vi "RT Main.vi"() -> ()   [LabVIEW 2011]
uses:
  RT/TypeDefs/Recipe Engine Commands.ctl
  RT/TypeDefs/Recipe Engine States.ctl
  <vilib>/Platform/TimedLoop/XDataNode/timing_clust.ctl
  <vilib>/Platform/TimedLoop/XDataNode/nitl_modes.ctl
  <vilib>/Platform/TimedLoop/XDataNode/wakeup.ctl
  RT/TypeDefs/Recipe Phase.ctl
  <vilib>/FPGAPlugInAG/cRIO-9074/niLvFpga_Open_cRIO-9074.vi
  <vilib>/rvi/interface/common/dynamic/niFpgaDynamicAddResources.vi
  <vilib>/FPGAPlugInAG/Dynamic/niLvFpga_Close_Dynamic.vi
  <vilib>/Platform/TimedLoop/XDataNode/loadnilvce.vi
  <vilib>/addons/control/pid/pid.llb/PID (DBL).vi
  <vilib>/Platform/TimedLoop/XDataNode/XDataNode.xnode
  <vilib>/rvi/interface/nirviOpenFPGA/nirviOpenFPGA.xnode
  FPGA Bitfiles/Bioreactor_FPGATarget_FPGAMain_8731874D.lvbitx
  FPGA Main.vi
  <vilib>/rvi/interface/nirviCloseFPGA/nirviCloseFPGA.xnode
  <vilib>/addons/control/pid/NI_PID_pid.lvlib
  <vilib>/Platform/TimedLoop/XDataNode/XDNodeRunTimeDep.lvlib
panel:
  out "FPGA State":enum16{"Normal Operation", "Safe State"}(ring)
  out "error out":errorcluster
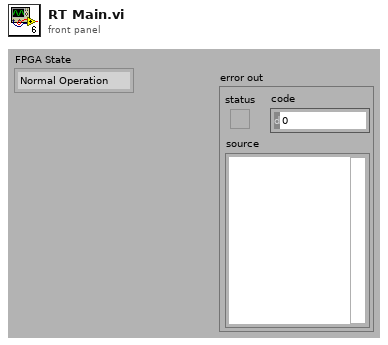
[diagram p1: front panel]
types:
  T1 = typedef "Recipe Engine Commands.ctl" = enum16{"Run Recipe", "Abort Recipe", "Exit"}
  T2 = typedef "Recipe Engine States.ctl" = enum16{"Initialize", "Wait for Cmd", "Load Phase", "Run Phase", "Exit"}
  T3 = typedef "XDNodeRunTimeDep.lvlib/timing_clust.ctl" = cluster{"Expected End [f-1]":u64, "Actual End [f-1]":u64, "Finished Late? [f-1]":bool, "Expected End [i-1]":u64, "Actual End [i-1]":u64, "Finished Late? [i-1]":bool, "Expected Start [i]":u64, "Actual Start [i]":u64, "Expected Start [f]":u64, "Actual Start [f]":u64, "Source Name":string, "Structure Name":string, "Period":i64, "Deadline":i64, "Offset":i64, "Start":i64, "Priority":i32, "Timeout":i32, "Mode":T4, "Wakeup Reason":T5, "Error":errorcluster, "Source Type":string, "Secondary Source Type":string, "Global End Time":u64, "Global Start Time":u64, "Frame Duration":u64, "Iteration Duration":u64, "Assigned CPU":i32, "I/O Scan Engine Mode":u32}
  T4 = typedef "XDNodeRunTimeDep.lvlib/nitl_modes.ctl" = enum32{"No Change", "Process missed periods, maintain original phase", "Discard missed periods, maintain original phase", "Process missed periods, ignore original phase", "Discard missed periods, ignore original phase"}
  T5 = typedef "XDNodeRunTimeDep.lvlib/wakeup.ctl" = enum32{"Normal", "Aborted", "Asynchronous wakeup", "Timing source error", "Timed loop error", "Timeout"}
  T6 = typedef "Recipe Phase.ctl" = cluster{"Temp Setpoint":dbl, "pH Setpoint":dbl, "Agitation ON":bool, "Intake ON":bool, "Waste ON":bool, "Time (s)":i32}
  T7 = cluster{"proportional gain (Kc)":dbl, "integral time (Ti, min)":dbl, "derivative time (Td, min)":dbl}
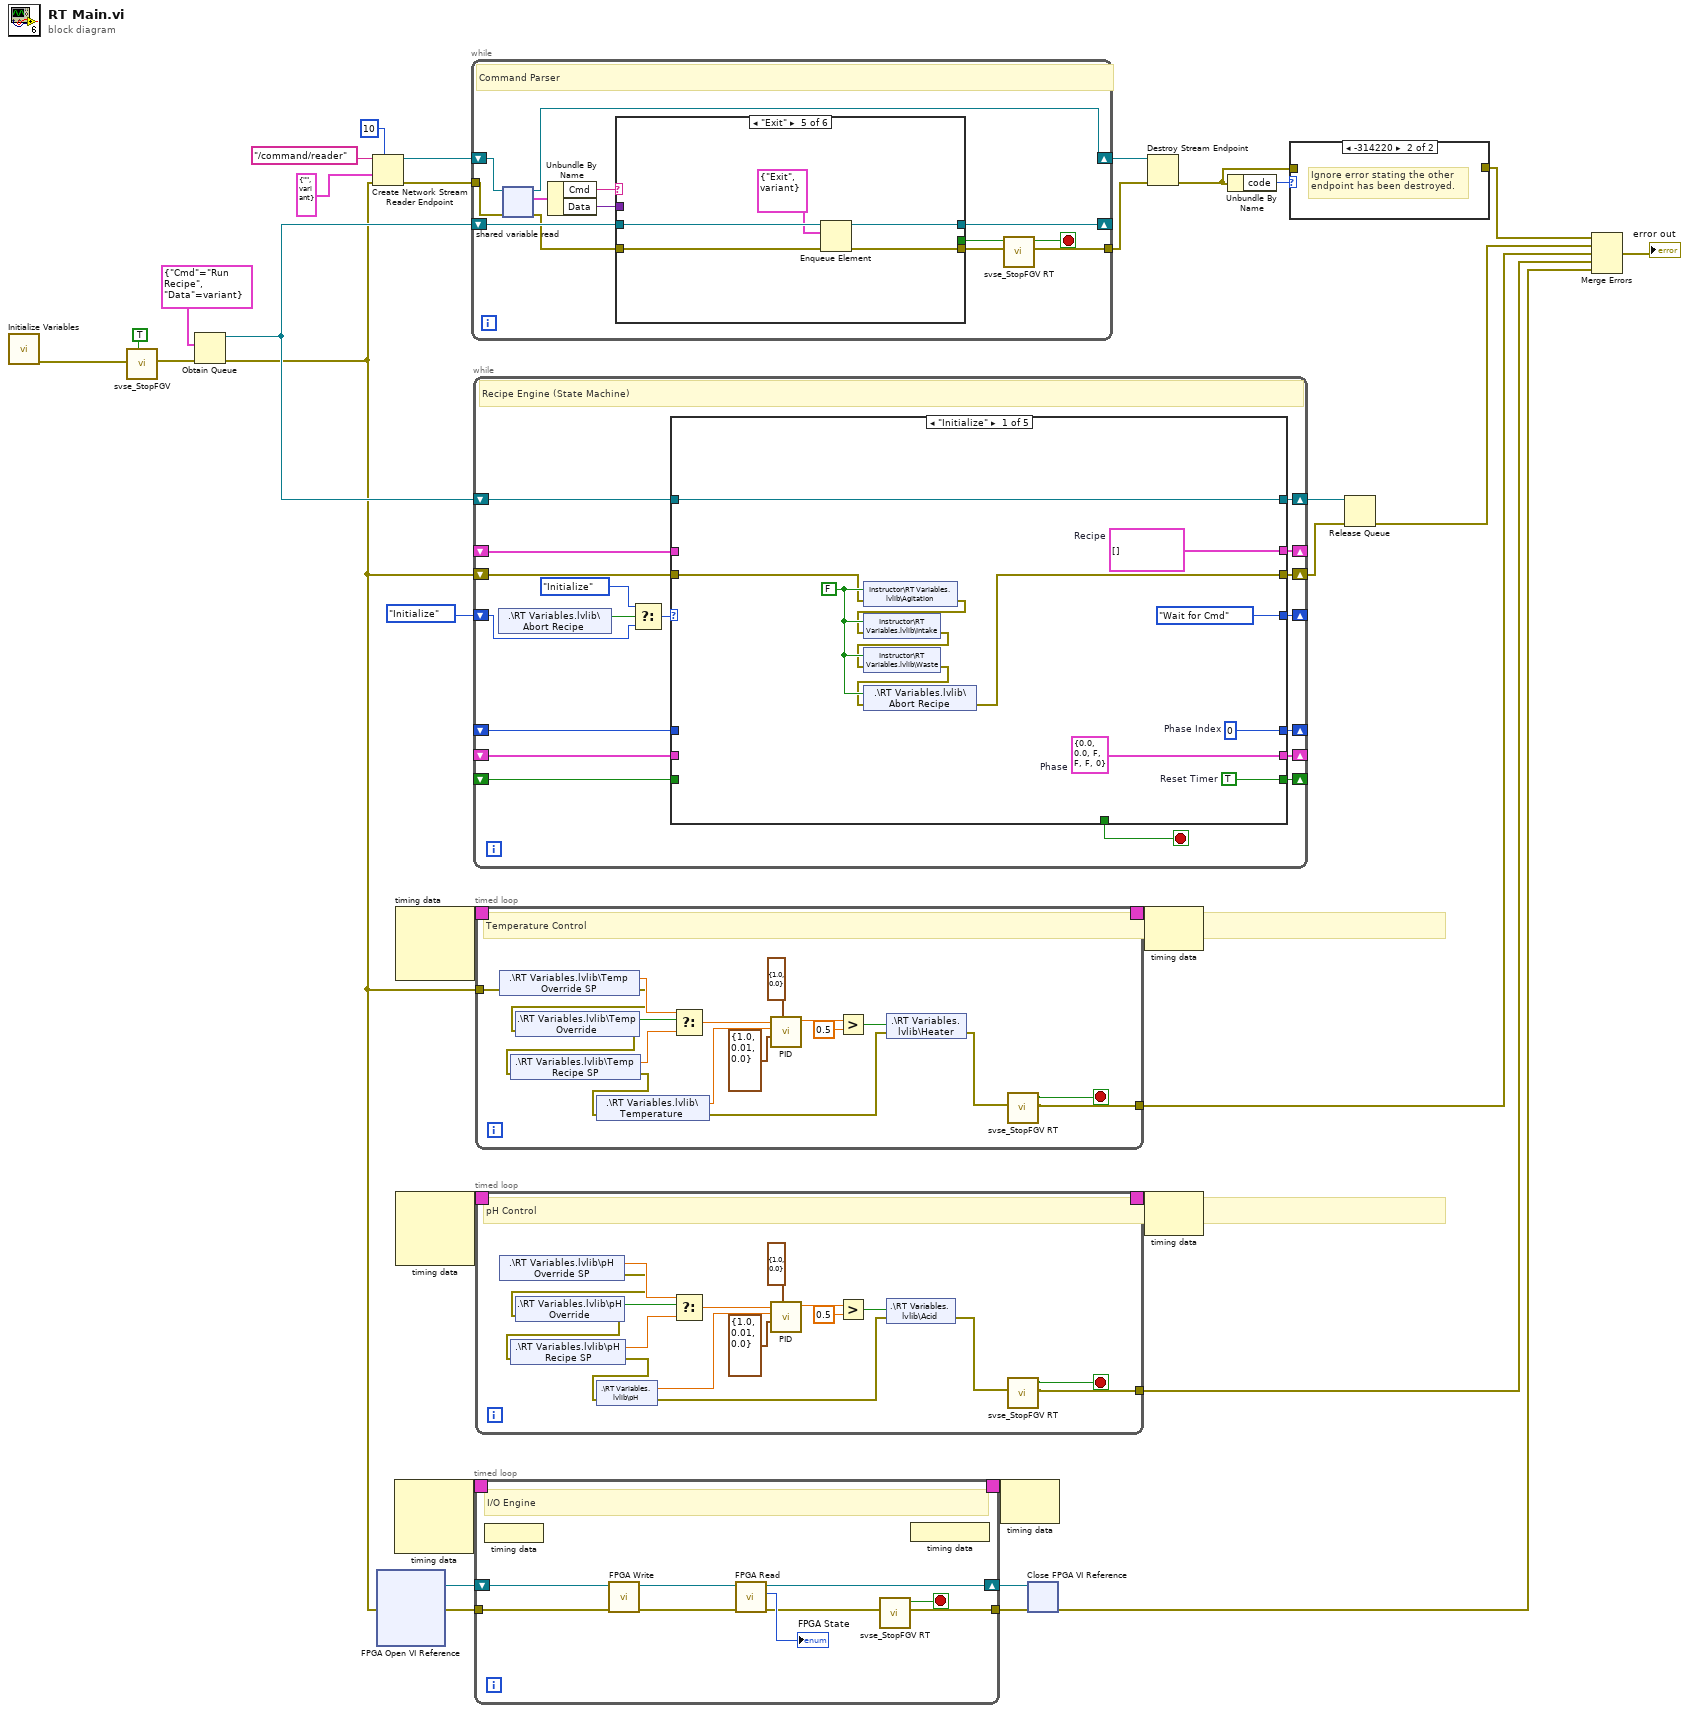
[diagram p0: block diagram]
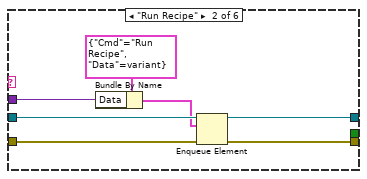
[diagram p4: hidden frame]
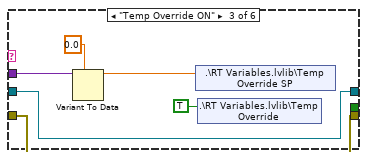
[diagram p5: hidden frame]
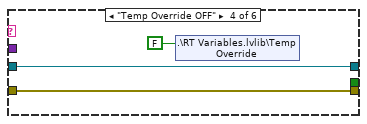
[diagram p6: hidden frame]
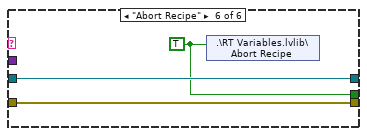
[diagram p7: hidden frame]
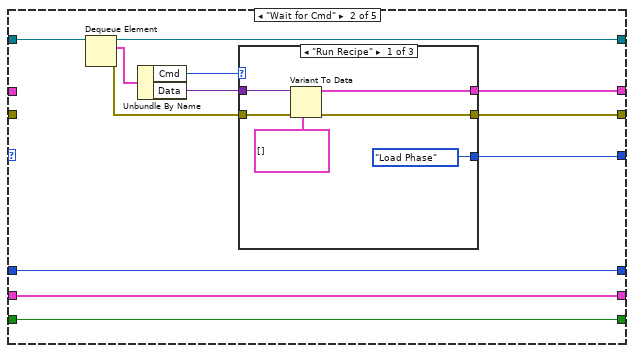
[diagram p8: hidden frame]
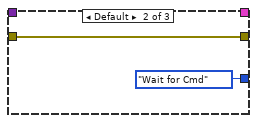
[diagram p9: hidden frame]
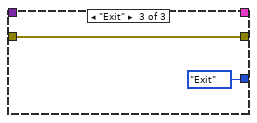
[diagram p10: hidden frame]
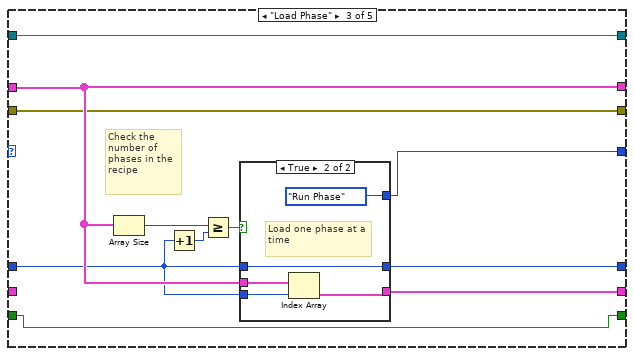
[diagram p11: hidden frame]
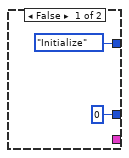
[diagram p12: hidden frame]
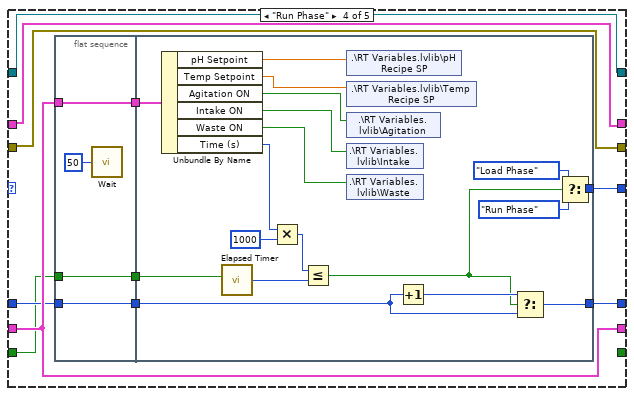
[diagram p13: hidden frame]
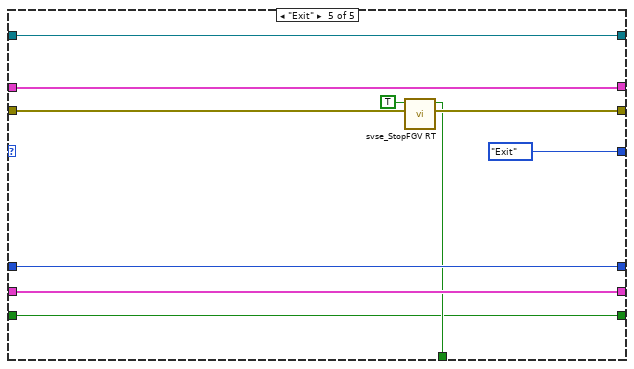
[diagram p14: hidden frame]
diagram:
  n1 = call "Initialize Variables.vi"() -> ("error out"=w9:errorcluster)  [unwired: 11 in]
  n2 = call "svse_StopFGV.vi"("Reset (F)"=TRUE, "error in"=w9) -> ("error out"=w8:errorcluster)  [unwired: 8 in, 1 out]
  n3 = Obtain Queue(element data type=cluster{"Cmd":T1, "Data":variant} {"Cmd"=enum."Run Recipe", "Data"=variant}, error in (no error)=w8) -> (queue out=w27:refnum<queue>, error out=w20:errorcluster)  [unwired: 3 in, 1 out]
  n4 = Create Network Stream Reader Endpoint(7:10 ("reader buffer size"), 8:w20, 9:cluster{"Cmd":string, "Data":variant} {"Cmd"="", "Data"=variant}, 11:"/command/reader" ("reader url")) -> (0:w28:errorcluster, 3:w30:refnum<k21>)  [unwired: 2 in]
  n5 = xnode "FPGA Open VI Reference"("error in"=w20) -> ("FPGA VI Reference Out"=w17:refnum<k20>, "error out"=w16:errorcluster)  [unwired: 1 in]
  n6 = node-c288() -> (w22:T3)  [unwired: 3 in]
  n7 = node-c288() -> (w26:T3)  [unwired: 3 in]
  n8 = node-c288() -> (w14:T3)  [unwired: 3 in]
  n9 = while {
    shift-right: [w35] -> w15
    shift-left: w30 -> [w43]
    shift-right: [w42] -> _
    shift-left: w27 -> [w44]
    tunnel: w28 -> [w41]
    tunnel: [w36] -> w4
    stop <- w38 stop-if-true
    # "Command Parser"
    n10 = shared-variable-read(w43, w41) -> (w35:refnum<k21>, w40:errorcluster, w47:cluster{"Cmd":string, "Data":variant})  [unwired: 1 in, 1 out]
    n11 = Unbundle By Name(w47) -> ("Cmd"=w46:string, "Data"=w45:variant)
    n12 = case shown="\"Exit\"" w46 {
      tunnel: w45 -> [_ w54 w62 _ _ _]
      tunnel: w44 -> [w49 w56 w60 w65 w70 w73]
      tunnel: [w49 w52 w60 w65 w68 w73] -> w42
      tunnel: w40 -> [w48 w51 w57 w63 w69 w72]
      tunnel: [w48 w50 w57 w63 w66 w72] -> w39
      tunnel: [_ _ _ _ _ w71] -> w37
      frame Default {
      }
      frame "Run Recipe" {
        n13 = Bundle By Name(cluster=cluster{"Cmd":T1, "Data":variant} {"Cmd"=enum."Run Recipe", "Data"=variant}, "Data"=w54) -> (w53:cluster{"Cmd":T1, "Data":variant})
        n14 = Enqueue Element(queue=w56, element=w53, error in (no error)=w51) -> (queue out=w52:refnum<queue>, error out=w50:errorcluster)  [unwired: 1 in, 1 out]
      }
      frame "Temp Override ON" {
        n15 = Variant To Data(type=0.0, Variant=w62) -> (data=w59:dbl)  [unwired: 1 in, 1 out]
        n16 = shared-variable ".\\RT Variables.lvlib\\Temp Override SP"(w59) -> ()  [unwired: 1 in, 1 out]
        n17 = shared-variable ".\\RT Variables.lvlib\\Temp Override"(TRUE ("Temp Override")) -> ()  [unwired: 1 in, 1 out]
      }
      frame "Temp Override OFF" {
        n18 = shared-variable ".\\RT Variables.lvlib\\Temp Override"(FALSE ("Temp Override")) -> ()  [unwired: 1 in, 1 out]
      }
      frame "Exit" {
        n19 = Enqueue Element(queue=w70, element=cluster{"Cmd":T1, "Data":variant} {"Cmd"=enum."Exit", "Data"=variant}, error in (no error)=w69) -> (queue out=w68:refnum<queue>, error out=w66:errorcluster)  [unwired: 1 in, 1 out]
      }
      frame "Abort Recipe" {
        w71 = TRUE ("Abort")
        n20 = shared-variable ".\\RT Variables.lvlib\\Abort Recipe"(w71) -> ()  [unwired: 1 in, 1 out]
      }
    }
    n21 = call "svse_StopFGV RT.vi"("error in"=w39, "User stop? (F)"=w37) -> ("error out"=w36:errorcluster, "Stop?"=w38:bool)  [unwired: 8 in]
  }
  n22 = while "Recipe" {
    shift-right: [w90] -> w1
    shift-left: w27 -> [w91]
    shift-right: [w89] -> _
    shift-left: _ -> [w87]
    shift-right: [w88] -> _
    shift-left: Recipe_Engine_States."Initialize" ("Enum") -> [w76]
    shift-right: [w85] -> _
    shift-left: _ -> [w86]
    shift-right: [w84] -> _
    shift-left: _ -> [w83]
    shift-right: [w82] -> _
    shift-left: _ -> [w81]
    shift-right: [w80] -> w3
    shift-left: w20 -> [w79]
    stop <- w74 stop-if-true
    # "Recipe Engine (State Machine)"
    n23 = shared-variable ".\\RT Variables.lvlib\\Abort Recipe"() -> (w78:bool)  [unwired: 1 in, 1 out]
    n24 = Select(t=Recipe_Engine_States."Initialize" ("Enum"), s=w78, f=w76) -> (s? t:f=w75:T2)
    n25 = case shown="\"Initialize\"" w75 {
      tunnel: w91 -> [w98 w115 w136 w150 w186]
      tunnel: [w98 w114 w136 w150 w186] -> w90
      tunnel: [w103 w110 w134 w149 w185] -> w89
      tunnel: [Recipe_Engine_States."Wait for Cmd" ("Enum") w109 w131 w151 Recipe_Engine_States."Exit" ("Enum")] -> w88
      tunnel: w87 -> [_ _ w134 w149 w185]
      tunnel: w86 -> [_ w104 w128 w152 w183]
      tunnel: [w101 w104 w130 w153 w183] -> w85
      tunnel: [w102 w108 w133 w154 w182] -> w84
      tunnel: w83 -> [_ w108 _ w154 w182]
      tunnel: [w100 w105 w126 _ w177] -> w82
      tunnel: w81 -> [_ w105 w126 w148 w177]
      tunnel: [w92 w106 w129 w147 w180] -> w80
      tunnel: w79 -> [w96 _ w129 w147 w181]
      tunnel: [_ _ _ _ w179] -> w74
      frame "Initialize" {
        w97 = FALSE ("Agitation")
        w100 = TRUE  # Reset Timer
        w101 = 0  # Phase Index
        w102 = T6 {"Temp Setpoint"=0.0, "pH Setpoint"=0.0, "Agitation ON"=FALSE, "Intake ON"=FALSE, "Waste ON"=FALSE, "Time (s)"=0}  # Phase
        w103 = T6[] []  # Recipe
        n26 = shared-variable "Instructor\\RT Variables.lvlib\\Agitation"(w97, error in=w96) -> (error out=w95:errorcluster)
        n27 = shared-variable "Instructor\\RT Variables.lvlib\\Intake"(w97, error in=w95) -> (error out=w94:errorcluster)
        n28 = shared-variable "Instructor\\RT Variables.lvlib\\Waste"(w97, error in=w94) -> (error out=w93:errorcluster)
        n29 = shared-variable ".\\RT Variables.lvlib\\Abort Recipe"(w97, error in=w93) -> (error out=w92:errorcluster)
      }
      frame "Wait for Cmd" {
        n30 = Dequeue Element(queue=w115) -> (queue out=w114:refnum<queue>, element=w113:cluster{"Cmd":T1, "Data":variant}, error out=w107:errorcluster)  [unwired: 2 in, 1 out]
        n31 = Unbundle By Name(w113) -> ("Cmd"=w112:T1, "Data"=w111:variant)
        n32 = case shown="\"Run Recipe\"" w112 {
          tunnel: w111 -> [w121 _ _]
          tunnel: [w119 _ _] -> w110
          tunnel: [Recipe_Engine_States."Load Phase" ("Enum") Recipe_Engine_States."Wait for Cmd" ("Enum") Recipe_Engine_States."Exit" ("Enum")] -> w109
          tunnel: w107 -> [w117 w122 w124]
          tunnel: [w116 w122 w124] -> w106
          frame "Run Recipe" {
            n33 = Variant To Data(error in=w117, type=T6[] [], Variant=w121) -> (data=w119:T6[], error out=w116:errorcluster)
          }
          frame Default {
          }
          frame "Exit" {
          }
        }
      }
      frame "Load Phase" {
        # "Check the number of phases in the recipe"
        n34 = Array Size(array=w134) -> (size(s)=w135:i32)
        n35 = Increment(x=w128) -> (x+1=w127:i32)
        n36 = Greater Or Equal?(x=w135, y=w127) -> (x >= y?=w132:bool)
        n37 = case shown="True" w132 {
          tunnel: w134 -> [_ w143]
          tunnel: [_ w142] -> w133
          tunnel: w128 -> [_ w141]
          tunnel: [Recipe_Engine_States."Initialize" ("Enum") Recipe_Engine_States."Run Phase" ("Enum")] -> w131
          tunnel: w128 -> [_ w139]
          tunnel: [0 ("Current Phase") w139] -> w130
          frame False {
          }
          frame True {
            # "Load one phase at a time"
            n38 = Index Array "Index Array"(array=w143, index=w141) -> (element=w142:T6)
          }
        }
      }
      frame "Run Phase" {
        n39 = flat-sequence {
          tunnel: w148 -> [w156]
          tunnel: w152 -> [w157]
          tunnel: w154 -> [w158]
          tunnel: [w158] -> w146
          tunnel: [w157] -> w145
          tunnel: [w156] -> w144
          tunnel: [w175] -> w153
          tunnel: [w173] -> w151
          tunnel: w146 -> [w176]
          tunnel: w145 -> [w174]
          tunnel: w144 -> [w172]
          frame #0 {
            n40 = call "Wait"("Count(uSec)"=u32 50) -> ()  [unwired: 1 out]
          }
          frame #1 {
            n41 = Unbundle By Name(w176) -> ("pH Setpoint"=w163:dbl, "Temp Setpoint"=w162:dbl, "Agitation ON"=w161:bool, "Intake ON"=w160:bool, "Waste ON"=w159:bool, "Time (s)"=w167:i32)
            n42 = call "Elapsed Timer.vi"("Reset Timer"=w172) -> ("Elapsed Time (ms)"=w164:u32)  [unwired: 10 in]
            n43 = Multiply(x=w167, y=1000) -> (x*y=w165:i32)
            n44 = Less Or Equal?(x=w165, y=w164) -> (x <= y?=w168:bool)
            n45 = shared-variable ".\\RT Variables.lvlib\\pH Recipe SP"(w163) -> ()  [unwired: 1 in, 1 out]
            n46 = shared-variable ".\\RT Variables.lvlib\\Temp Recipe SP"(w162) -> ()  [unwired: 1 in, 1 out]
            n47 = shared-variable ".\\RT Variables.lvlib\\Agitation"(w161) -> ()  [unwired: 1 in, 1 out]
            n48 = shared-variable ".\\RT Variables.lvlib\\Intake"(w160) -> ()  [unwired: 1 in, 1 out]
            n49 = shared-variable ".\\RT Variables.lvlib\\Waste"(w159) -> ()  [unwired: 1 in, 1 out]
            n50 = Increment(x=w174) -> (x+1=w171:i32)
            n51 = Select(t=w171, s=w168, f=w174) -> (s? t:f=w175:i32)
            n52 = Select(t=Recipe_Engine_States."Load Phase" ("Enum"), s=w168, f=Recipe_Engine_States."Run Phase" ("Enum")) -> (s? t:f=w173:T2)
          }
        }
      }
      frame "Exit" {
        n53 = call "svse_StopFGV RT.vi"("error in"=w181, "User stop? (F)"=TRUE) -> ("error out"=w180:errorcluster, "Stop?"=w179:bool)  [unwired: 8 in]
      }
    }
  }
  n54 = timed-loop "I/O Engine" {
    timing: w22 -> [_]
    timing-out: [_] -> w21
    tunnel: w16 -> [w195]
    tunnel: [w188] -> w19
    shift-right: [w191] -> w18
    shift-left: w17 -> [w190]
    stop <- w187 stop-if-true
    # "I/O Engine"
    n55 = node-c288() -> ()  [unwired: 1 in]
    n56 = call "FPGA Write.vi"("error in"=w195, "FPGA VI Reference In"=w190) -> ("error out"=w194:errorcluster, "FPGA VI Reference Out"=w192:refnum<k20>)  [unwired: 8 in]
    n57 = call "FPGA Read.vi"("error in (no error)"=w194, "FPGA VI Reference In"=w192) -> ("error out"=w189:errorcluster, "FPGA State"=→"FPGA State":enum16{"Normal Operation", "Safe State"}, "FPGA VI Reference Out"=w191:refnum<k20>)  [unwired: 6 in]
    n58 = call "svse_StopFGV RT.vi"("error in"=w189) -> ("error out"=w188:errorcluster, "Stop?"=w187:bool)  [unwired: 9 in]
    n59 = node-c288() -> ()  [unwired: 1 out]
  }
  n60 = timed-loop "Temp Ctrl" {
    timing: w26 -> [_]
    timing-out: [_] -> w25
    tunnel: w20 -> [w202]
    tunnel: [w208] -> w23
    stop <- w207 stop-if-true
    # "Temperature Control"
    n61 = shared-variable ".\\RT Variables.lvlib\\Temp Override SP"(error in=w202) -> (w204:dbl, error out=w201:errorcluster)
    n62 = shared-variable ".\\RT Variables.lvlib\\Temp Override"(error in=w201) -> (w205:bool, error out=w200:errorcluster)
    n63 = shared-variable ".\\RT Variables.lvlib\\Temp Recipe SP"(error in=w200) -> (w203:dbl, error out=w199:errorcluster)
    n64 = shared-variable ".\\RT Variables.lvlib\\Temperature"(error in=w199) -> (w210:dbl, error out=w198:errorcluster)
    n65 = Select(t=w204, s=w205, f=w203) -> (s? t:f=w215:dbl)
    n66 = call-poly <vilib>:"PID.vi"("output range"=cluster{"output high":dbl, "output low":dbl} {"output high"=1.0, "output low"=0.0}, "PID gains"=T7 {"proportional gain (Kc)"=1.0, "integral time (Ti, min)"=0.01, "derivative time (Td, min)"=0.0}, "process variable"=w210, "setpoint"=w215) -> ("output"=w212:dbl)  [unwired: 6 in, 1 out]
    n67 = Greater?(x=w212, y=0.5) -> (0:w209:bool)
    n68 = shared-variable ".\\RT Variables.lvlib\\Heater"(w209, error in=w198) -> (error out=w206:errorcluster)
    n69 = call "svse_StopFGV RT.vi"("error in"=w206) -> ("error out"=w208:errorcluster, "Stop?"=w207:bool)  [unwired: 9 in]
  }
  n70 = timed-loop "Temp Ctrl" {
    timing: w14 -> [_]
    timing-out: [_] -> w13
    tunnel: [w227] -> w11
    stop <- w226 stop-if-true
    # "pH Control"
    n71 = shared-variable ".\\RT Variables.lvlib\\pH Override SP"() -> (w223:dbl, error out=w221:errorcluster)  [unwired: 1 in]
    n72 = shared-variable ".\\RT Variables.lvlib\\pH Override"(error in=w221) -> (w224:bool, error out=w220:errorcluster)
    n73 = shared-variable ".\\RT Variables.lvlib\\pH Recipe SP"(error in=w220) -> (w222:dbl, error out=w219:errorcluster)
    n74 = shared-variable ".\\RT Variables.lvlib\\pH"(error in=w219) -> (w229:dbl, error out=w218:errorcluster)
    n75 = Select(t=w223, s=w224, f=w222) -> (s? t:f=w234:dbl)
    n76 = call-poly <vilib>:"PID.vi"("output range"=cluster{"output high":dbl, "output low":dbl} {"output high"=1.0, "output low"=0.0}, "PID gains"=T7 {"proportional gain (Kc)"=1.0, "integral time (Ti, min)"=0.01, "derivative time (Td, min)"=0.0}, "process variable"=w229, "setpoint"=w234) -> ("output"=w231:dbl)  [unwired: 6 in, 1 out]
    n77 = Greater?(x=w231, y=0.5) -> (0:w228:bool)
    n78 = shared-variable ".\\RT Variables.lvlib\\Acid"(w228, error in=w218) -> (error out=w225:errorcluster)
    n79 = call "svse_StopFGV RT.vi"("error in"=w225) -> ("error out"=w227:errorcluster, "Stop?"=w226:bool)  [unwired: 9 in]
  }
  n80 = node-c288(w21) -> ()  [unwired: 1 out]
  n81 = xnode "Close FPGA VI Reference"("FPGA VI Reference In"=w18, "error in"=w19) -> ("error out"=w12:errorcluster)
  n82 = node-c288(w25) -> ()  [unwired: 1 out]
  n83 = node-c288(w13) -> ()  [unwired: 1 out]
  n84 = Destroy Stream Endpoint(8:w4, 11:w15) -> (0:w6:errorcluster)
  n85 = Unbundle By Name(w6) -> ("code"=w7:i32)
  n86 = case shown="-314220" w7 {
    tunnel: w6 -> [w237 _]
    tunnel: [w237 _] -> w5
    frame 0, Default {
    }
    frame -314220 {
      # "Ignore error stating the other\nendpoint has been destroyed."
    }
  }
  n87 = Release Queue(queue=w1, error in (no error)=w3) -> (error out=w2:errorcluster)  [unwired: 1 in, 2 out]
  n88 = Merge Errors(w5, w2, w23, w11, w12) -> (→"error out":errorcluster)
